vi "DO Read Line.vi"(7 "Value":u16, 8 "error in (no error)":errorcluster caption="错误输入（无错误）", 9 "Line":u16, 10 "Port":u16, 11 "CardNumber":u16) -> (0 "error out":errorcluster caption="错误输出", 3 "function return":i16, 5 "Value out":u16)   [LabVIEW 2014, in "Adlink IO.lvlib"]
doc: "I16 __stdcall DO_ReadLine(U16 CardNumber, U16 Port, U16 Line, U16 *Value);"
uses:
  Adlink IO.lvlib
  PCI-Dask.dll
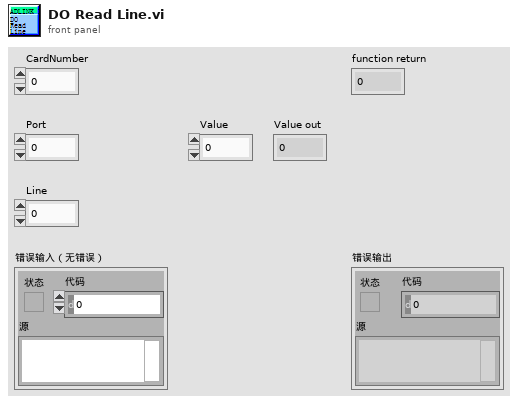
[diagram p1: front panel]
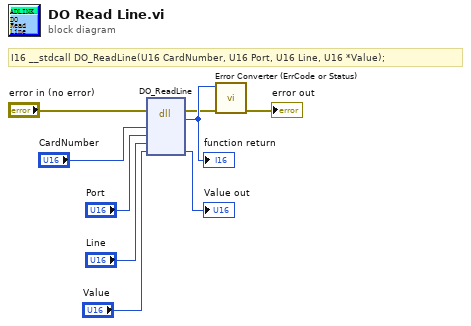
[diagram p0: block diagram]
diagram:
  # "I16 __stdcall DO_ReadLine(U16 CardNumber, U16 Port, U16 Line, U16 *Value);"
  n1 = dll-call lib="PTH2sabs D中山贴膜机最最终极版3纬创贴膜机SubViADLINKIOADLINK IO demo\tAdlink IO\nPCI-Dask.*" fn="DO_ReadLine"(error in="error in (no error)", "CardNumber"="CardNumber", "Port"="Port", "Line"="Line", "Value"="Value") -> (error out=w2:errorcluster, w9:i16, "Value"=→"Value out":u16)  [unwired: 5 in, 1 out]
  "function return" <- w9
  n2 = call "Error Converter (ErrCode or Status).vi"("error in (no error)"=w2, "error code"=w9) -> ("error out"=→"error out":errorcluster)  [unwired: 9 in]
